vi "SCELTA LINEA.vi"(10 "Scelta inverter":T1(ring)=enum."INVERTER 2 [75kW]", 11 "Vn [V]":dbl) -> (3 "Array":bool[](array[boolean]))   [LabVIEW 2019]
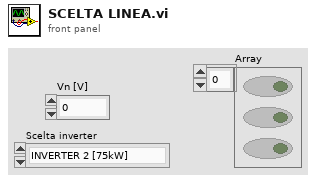
[diagram p1: front panel]
types:
  T1 = enum32{"No Selection", "INVERTER 1 [7,5kW]", "INVERTER 2 [75kW]", "INVERTER 3"}
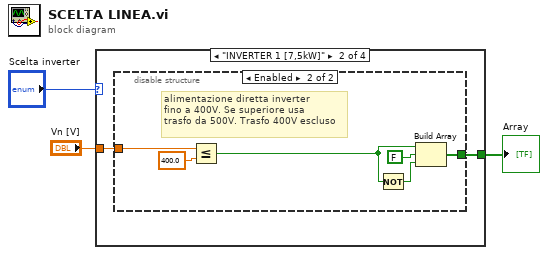
[diagram p0: block diagram]
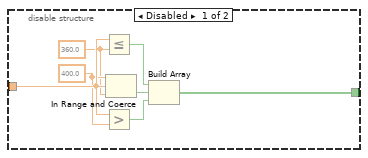
[diagram p3: hidden frame]
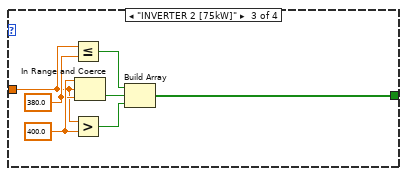
[diagram p4: hidden frame]
diagram:
  n1 = case shown="\"INVERTER 1 [7,5kW]\"" "Scelta inverter" {
    tunnel: "Vn [V]" -> [_ w5 w20 _]
    tunnel: [_ w4 w19 _] -> w2
    frame "No Selection", Default {
    }
    frame "INVERTER 1 [7,5kW]" {
      n2 = disable-structure shown="Enabled" {
        disable-tunnel: w5 -> [w12 w16]
        disable-tunnel: [w11 w17] -> w4
        frame Disabled {
          w7 = 400.0 ("upper limit")
          w6 = 360.0 ("y")
          n3 = Less Or Equal?(x=w12, y=w6) -> (x <= y?=w8:bool)
          n4 = Greater?(x=w12, y=w7) -> (0:w10:bool)
          n5 = In Range and Coerce(upper limit=w7, x=w12, lower limit=w6) -> (In Range?=w9:bool)  [unwired: 1 out]
          n6 = Build Array(w8, w9, w10) -> (w11:bool[])
        }
        frame Enabled {
          # "alimentazione diretta inverter\nfino a 400V. Se superiore usa\ntrasfo da 500V. Trasfo 400V escluso"
          n7 = Less Or Equal?(x=w16, y=400.0) -> (x <= y?=w13:bool)
          n8 = Not(x=w13) -> (.not. x?=w14:bool)
          n9 = Build Array(w13, FALSE ("element"), w14) -> (w17:bool[])
        }
      }
    }
    frame "INVERTER 2 [75kW]" {
      w22 = 400.0 ("upper limit")
      w21 = 380.0 ("y")
      n10 = Less Or Equal?(x=w20, y=w21) -> (x <= y?=w23:bool)
      n11 = Greater?(x=w20, y=w22) -> (0:w25:bool)
      n12 = In Range and Coerce(upper limit=w22, x=w20, lower limit=w21) -> (In Range?=w24:bool)  [unwired: 1 out]
      n13 = Build Array(w23, w24, w25) -> (w19:bool[])
    }
    frame "INVERTER 3" {
    }
  }
  "Array" <- w2
